vi "IntakeTeleOp.vi"(6 "Speed for intake":i32, 9 "Duration":i32, 10 "Retrieve":bool, 11 "Shoot":bool) -> ()   [LabVIEW 2015]
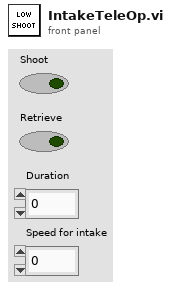
[diagram p1: front panel]
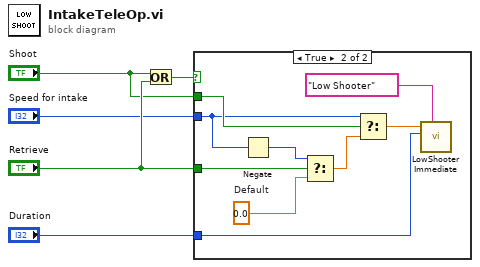
[diagram p0: block diagram]
diagram:
  n1 = Or(x="Shoot", y="Retrieve") -> (x .or. y?=w3:bool)
  n2 = case shown="True" w3 {
    tunnel: "Shoot" -> [_ w11]
    tunnel: "Retrieve" -> [_ w12]
    tunnel: "Speed for intake" -> [_ w7]
    tunnel: "Duration" -> [_ w13]
    frame False {
    }
    frame True {
      w6 = 0.0  # Default
      n3 = Negate(x=w7) -> (-x=w8:i32)
      n4 = Select(t=w8, s=w12, f=w6) -> (s? t:f=w10:dbl)
      n5 = Select(t=w7, s=w11, f=w10) -> (s? t:f=w9:dbl)
      n6 = call "LowShooter Immediate.vi"("Description"="Low Shooter", "Duration"=w13, "Setpoint"=w9) -> ()  [unwired: 8 in, 1 out]
    }
  }
